vi "helper_binaryRead.vi"() -> ()   [LabVIEW 2021]
uses:
  <vilib>/numeric/Random Number (Range) I64.vi
  <vilib>/numeric/sub_Random U32.vi
panel:
  out "size(s) 2":i32
  out "size(s)":i32
  out "Array":i32[](array[numeric])
  out "size (in bytes)":i64
  out "data":i16[](array[numeric])
  out "error out":errorcluster
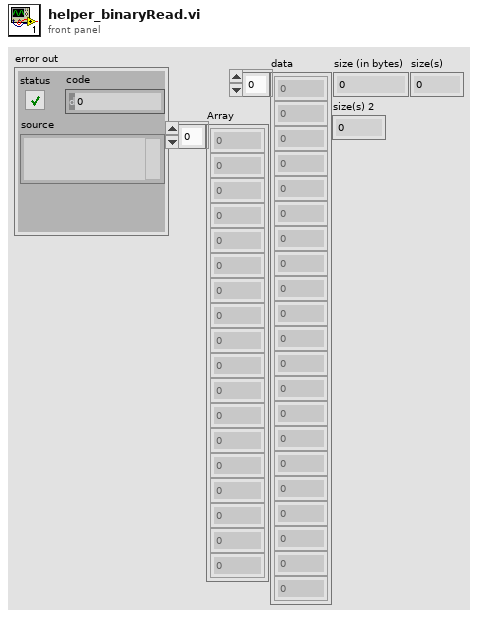
[diagram p1: front panel]
types:
  T1 = enum16{"big-endian, network order", "native, host order", "little-endian"}
  T2 = enum16{"open", "replace", "create", "open or create", "replace or create", "replace or create with confirmation"}
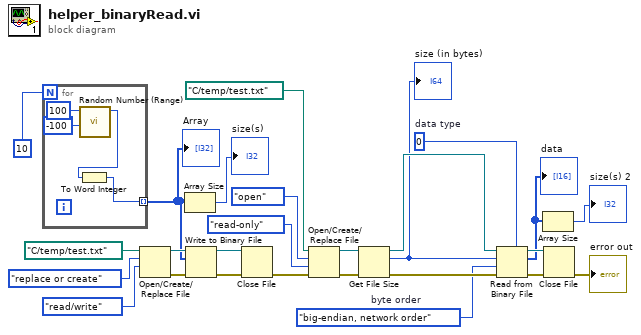
[diagram p0: block diagram]
diagram:
  w10 = T1."big-endian, network order"  # byte order
  w11 = i16 0  # data type
  n1 = for {
    N: 10 -> [_]
    tunnel: [w27] -> w1 mode=indexing
    n2 = call-poly <vilib>:"Random Number (Range).vi"("lower bound (-100)"=i64 -100, "upper bound (100)"=i64 100) -> ("number"=w28:i64)  [unwired: 9 in]
    n3 = To Word Integer(number=w28) -> (16bit integer=w27:i16)
  }
  "Array" <- w1
  n4 = Open/Create/Replace File(file path (use dialog)=path "C:/temp/test.txt", operation (0:open)=T2."replace or create", access (0:read/write)=enum16{"read/write", "read-only", "write-only"}."read/write") -> (refnum out=w22:refnum<file>, error out=w21:errorcluster)  [unwired: 3 in, 1 out]
  n5 = Array Size(array=w1) -> (size(s)=→"size(s)":i32)
  n6 = Write to Binary File(file (use dialog)=w22, data=w1, error in=w21) -> (refnum out=w20:refnum<file>, error out=w19:errorcluster)  [unwired: 3 in, 1 out]
  n7 = Close File(refnum=w20, error in=w19) -> (error out=w26:errorcluster)  [unwired: 1 out]
  n8 = Open/Create/Replace File(file path (use dialog)=path "C:/temp/test.txt", error in=w26, operation (0:open)=T2."open", access (0:read/write)=enum16{"read/write", "read-only", "write-only"}."read-only") -> (refnum out=w15:refnum<file>, error out=w16:errorcluster)  [unwired: 2 in, 1 out]
  n9 = Get File Size(file=w15, error in=w16) -> (refnum out=w13:refnum<file>, size (in bytes)=w2:i64, 0:w14:errorcluster)
  "size (in bytes)" <- w2
  n10 = Read from Binary File(5:w11, 8:w14, 9:w10, 10:w2, 11:w13) -> (0:w17:errorcluster, 2:w4:i16[], 3:w18:refnum<file>)  [unwired: 1 in, 1 out]
  "data" <- w4
  n11 = Array Size(array=w4) -> (size(s)=→"size(s) 2":i32)
  n12 = Close File(refnum=w18, error in=w17) -> (error out=→"error out":errorcluster)  [unwired: 1 out]
